vi "Loadcfg_writeslaveT.vi"(8 "error in":errorcluster, 11 "Data Cluster in":T2) -> (0 "error out":errorcluster, 3 "Data Cluster out":T2)   [LabVIEW 2017, in "Akwizycja.lvlib"]
uses:
  Akwizycja.lvlib
  <vilib>/Plasmionique/MB Master/MB_Master_Serial/MB_Master_Serial.lvclass
  D:/Program Files (x86)/National Instruments/LabVIEW 2017/vi.lib/Plasmionique/MB Master/MB_Master/MB_Master.lvclass
  <vilib>/Plasmionique/MB Master/MB Master.lvlib
  <vilib>/Utility/config.llb/NI_LVConfig.lvlib
panel:
  out "data":T1
  in  "Tx":T1
  # "Wejscie"
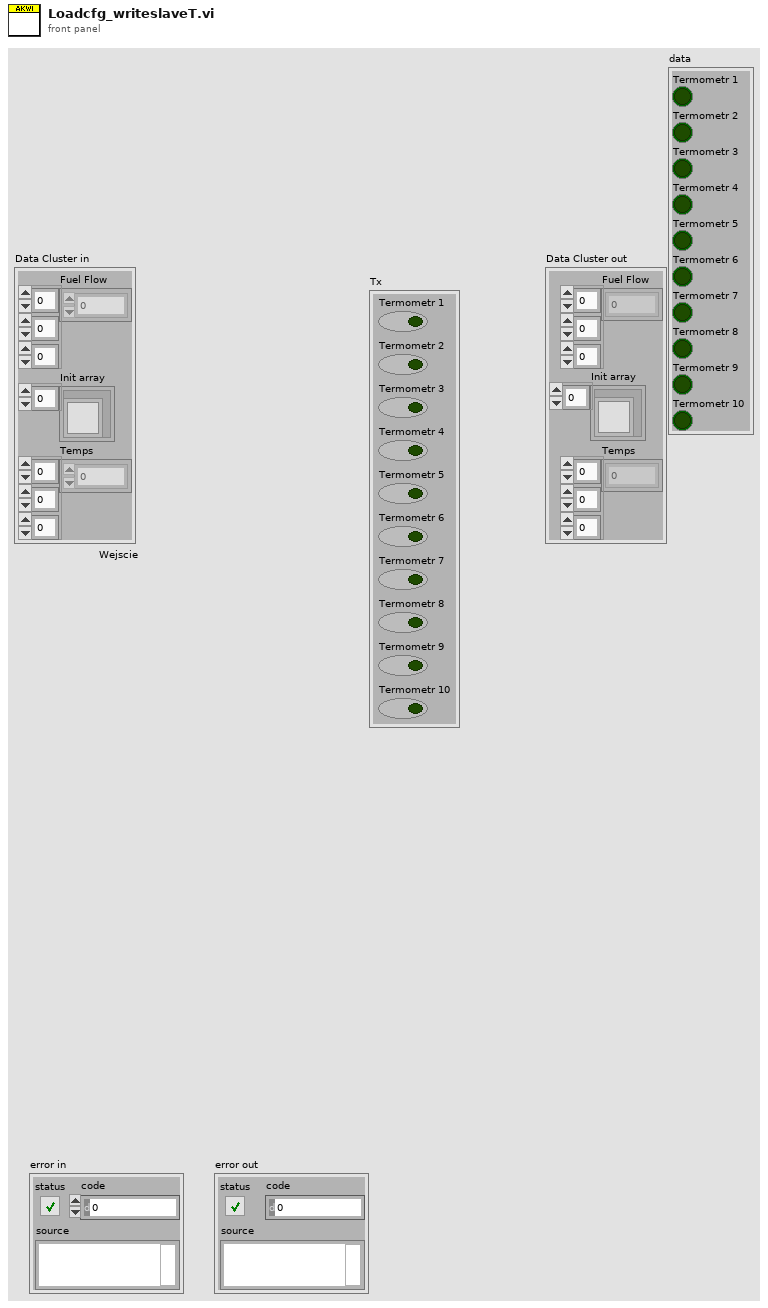
[diagram p1: front panel]
types:
  T1 = cluster{"Termometr 1":bool, "Termometr 2":bool, "Termometr 3":bool, "Termometr 4":bool, "Termometr 5":bool, "Termometr 6":bool, "Termometr 7":bool, "Termometr 8":bool, "Termometr 9":bool, "Termometr 10":bool}
  T2 = cluster{"Fuel Flow":dbl[][][], "Init array":refnum<class "MB_Master_Serial.lvclass">[], "Temps":dbl[][][]}
  T3 = typedef "NI_LVConfig.lvlib/Config Data RefNum.ctl" = refnum<k1>
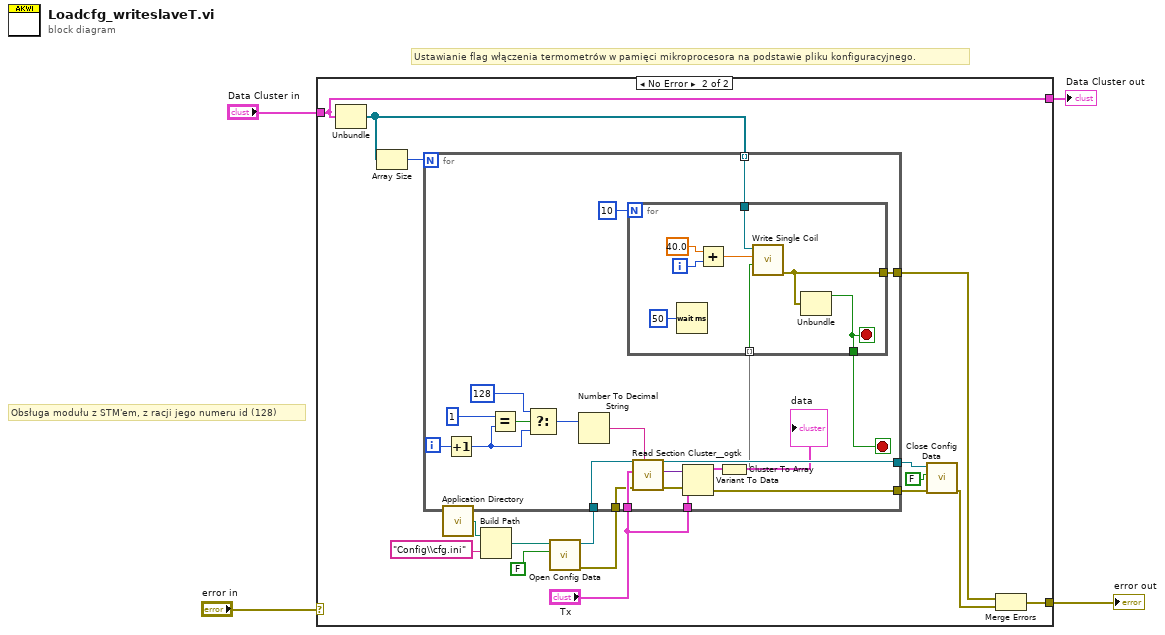
[diagram p0: block diagram]
diagram:
  # "Obsługa modułu z STM'em, z racji jego numeru id (128)"
  # "Ustawianie flag włączenia termometrów w pamięci mikroprocesora na podstawie pliku konfiguracyjnego."
  n1 = case shown="No Error" "error in" {
    selector: "error in" -> [w6 _]
    tunnel: [w6 w14] -> w4
    tunnel: "Data Cluster in" -> [w5 w8]
    tunnel: [w5 w8] -> w1
    frame Error {
    }
    frame No Error {
      n2 = Unbundle(w8) -> ("Init array"=w7:refnum<class "MB_Master_Serial.lvclass">[])  [unwired: 2 out]
      n3 = Array Size(array=w7) -> (size(s)=w9:i32)
      n4 = call <vilib>:"Application Directory.vi"() -> ("Application Directory"=w15:path)
      n5 = Build Path(base path=w15, name or relative path="Config\\cfg.ini") -> (appended path=w17:path)
      n6 = call <vilib>:"Open Config Data.vi"("create file if necessary (T)"=FALSE, "configuration file path"=w17) -> ("error out"=w13:errorcluster, "refnum"=w19:T3)  [unwired: 7 in, 1 out]
      n7 = for {
        N: w9 -> [_]
        tunnel: w19 -> [w43]
        tunnel: [w42] -> w20
        tunnel: [w40] -> w22
        tunnel: w7 -> [w25] mode=indexing
        tunnel: [w36] -> w12
        tunnel: "Tx" -> [w33]
        tunnel: "Tx" -> [w32]
        tunnel: w13 -> [w31]
        i -> [w24]
        stop <- w34 stop-if-true
        n8 = Increment(x=w24) -> (x+1=w23:i32)
        n9 = Equal?(x=1, y=w23) -> (x = y?=w28:bool)
        n10 = Select(t=128, s=w28, f=w23) -> (s? t:f=w26:i32)
        n11 = Number To Decimal String(number=w26) -> (decimal integer string=w30:string)  [unwired: 1 in]
        n12 = call <userlib>:"Read Section Cluster__ogtk.vi"("section (optional)"=w30, "error in (no error)"=w31, "Section Formatted Cluster Type"=w33, "refnum"=w43) -> ("error out"=w41:errorcluster, "Section Formatted Cluster"=w39:variant, "dup refnum"=w42:T3)  [unwired: 3 in, 2 out]
        n13 = Variant To Data(error in=w41, type=w32, Variant=w39) -> (data=w38:T1, error out=w40:errorcluster)
        "data" <- w38
        n14 = Cluster To Array(cluster=w38) -> (array=w35:bool[])
        n15 = for {
          N: 10 ("Numeric Control") -> [_]
          tunnel: w25 -> [w46]
          tunnel: [w47] -> w36
          tunnel: w35 -> [w48] mode=indexing
          tunnel: [w45] -> w34
          i -> [w49]
          stop <- w45 stop-if-true
          n16 = Wait (ms)(milliseconds to wait=u32 50) -> ()  [unwired: 1 out]
          n17 = Add(x=40.0, y=w49) -> (x+y=w50:dbl)
          n18 = call <vilib>:"Write Single Coil.vi"("value"=w48, "address"=w50, "MB session in"=w46) -> ("error out"=w47:errorcluster)  [unwired: 7 in, 1 out]
          n19 = Unbundle(w47) -> ("status"=w45:bool)  [unwired: 2 out]
        }
      }
      n20 = call <vilib>:"Close Config Data.vi"("error in (no error)"=w22, "write file if changed (T)"=FALSE, "refnum"=w20) -> ("error out"=w11:errorcluster)  [unwired: 7 in, 1 out]
      n21 = Merge Errors(w12, w11) -> (w14:errorcluster)
    }
  }
  "error out" <- w4
  "Data Cluster out" <- w1
